vi "Replace Special Characters.vi"(6 "Substitute":enum16{"char to special", "special to char"}(ring), 11 "Value":string) -> (3 "result string":string)   [LabVIEW 2020, in "Tree Map.lvlib"]
uses:
  Tree Map.lvlib
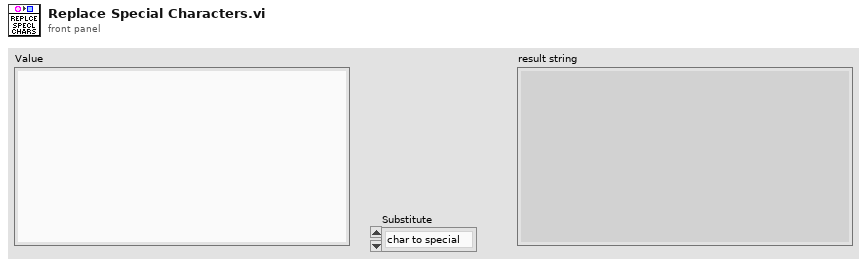
[diagram p1: front panel]
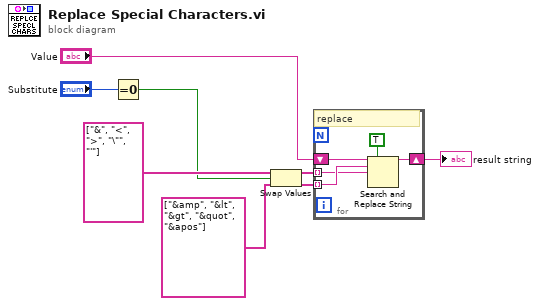
[diagram p0: block diagram]
diagram:
  n1 = Equal To 0?(x="Substitute") -> (x = 0?=w2:bool)
  n2 = Swap Values(12:string[] ["&", "<", ">", "\"", "'"] ("search string"), 13:w2, 14:string[] ["&amp", "&lt", "&gt", "&quot", "&apos"] ("replace string (\"\")")) -> (1:w6:string[], 3:w5:string[])
  n3 = for {
    shift-right: [w13] -> w8
    shift-left: "Value" -> [w12]
    tunnel: w5 -> [w10] mode=indexing
    tunnel: w6 -> [w9] mode=indexing
    # "replace"
    n4 = Search and Replace String(replace all?=TRUE ("replace all? (F)"), input string=w12, search string=w10, replace string=w9) -> (result string=w13:string)  [unwired: 4 in, 3 out]
  }
  "result string" <- w8
